vi "exp sequence exit logic.vi"(0 "PID exp exec in":T1, 7 "proceed":bool, 11 "exit":bool) -> (4 "stop loop":bool, 15 "Experimental Sequence":T2)   [LabVIEW 2019]
doc: "This subVI is just a convienience. It encapsulates some space filling exit logic for the initialization phase of the executive loop.\n\nPaul K Dixon\nP3600\nCSUSB Physics"
uses:
  typedefs/exp sequence.ctl
  typedefs/PID exec cluster.ctl
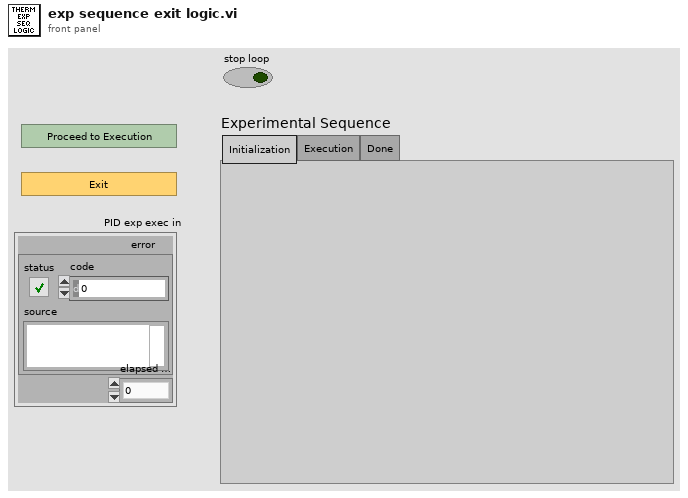
[diagram p1: front panel]
types:
  T1 = typedef "PID exec cluster.ctl" = cluster{"error":errorcluster, "elapsed time (s)":dbl}
  T2 = typedef "exp sequence.ctl" = enum32{"Initialization", "Execution", "Done"}
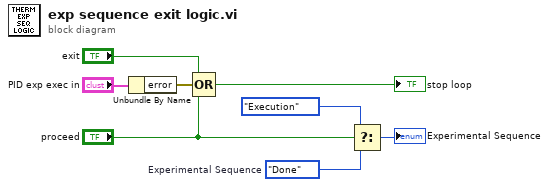
[diagram p0: block diagram]
diagram:
  w5 = exp_sequence."Done"  # Experimental Sequence
  n1 = Unbundle By Name("PID exp exec in") -> ("error"=w2:errorcluster)
  n2 = Compound Arithmetic op=OR("exit", w2, "proceed") -> (→"stop loop":bool)
  n3 = Select(t=exp_sequence."Execution" ("Experimental Sequence"), s="proceed", f=w5) -> (s? t:f=→"Experimental Sequence":T2)
